vi "MPM_Get_Wavelength_Senctivity_Data.vi"(8 "error in (no error)":errorcluster, 9 "channelNumber":i32, 10 "moduleNumber":i32, 11 ".NET Reference in":refnum<k24>) -> (0 "error out":errorcluster, 1 "offsetpower out":sgl[](array[numeric]), 2 "wavedata out":dbl[](array[numeric]), 3 "Reference out":refnum<k24>)   [LabVIEW 2017]
uses:
  LV_IL_Sample/DLL/InstrumentDLL.dll
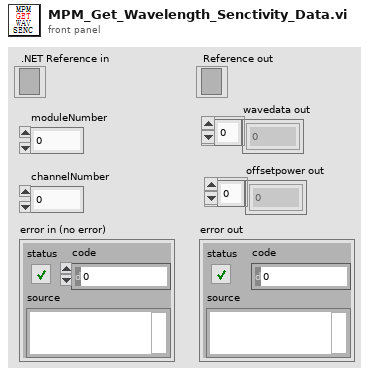
[diagram p1: front panel]
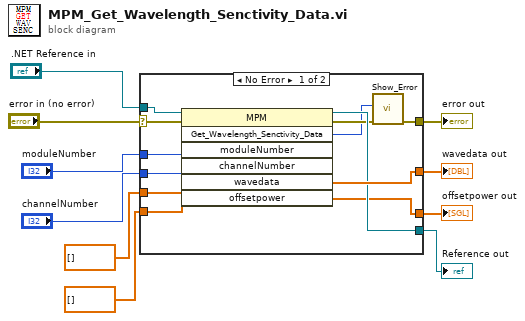
[diagram p0: block diagram]
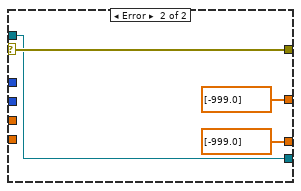
[diagram p2: hidden frame]
diagram:
  n1 = case shown="No Error" "error in (no error)" {
    selector: "error in (no error)" -> [w13 w26]
    tunnel: [w22 dbl[] [-999.0] ("wavedata")] -> w10
    tunnel: "channelNumber" -> [w21 _]
    tunnel: "moduleNumber" -> [w20 _]
    tunnel: ".NET Reference in" -> [w19 w25]
    tunnel: [w18 w25] -> w6
    tunnel: dbl[] [] ("wavedata") -> [w17 _]
    tunnel: [w15 w26] -> w4
    tunnel: sgl[] [] ("offsetpower") -> [w12 _]
    tunnel: [w11 sgl[] [-999.0] ("offsetpower")] -> w1
    frame No Error {
      n2 = invoke on="调用节点" class="MPM" method="Get_Wavelength_Senctivity_Data"(reference=w19, error in=w13, "moduleNumber"=w20, "channelNumber"=w21, "wavedata"=w17, "offsetpower"=w12) -> (reference out=w18:refnum<k24>, error out=w16:errorcluster, "Get_Wavelength_Senctivity_Data"=w14:i32, "wavedata"=w22:dbl[], "offsetpower"=w11:sgl[])  [unwired: 1 in, 2 out]
      n3 = call "Show_Error.vi"("error in (no error)"=w16, "Error"=w14) -> ("error out"=w15:errorcluster)  [unwired: 9 in]
    }
    frame Error {
    }
  }
  "wavedata out" <- w10
  "Reference out" <- w6
  "error out" <- w4
  "offsetpower out" <- w1
